vi "Factorial_Assignement.vi"() -> ()   [LabVIEW 2019]
panel:
  out "Result":i32
  in  "Numeric 2":i32
  # "Factorial Assignment"
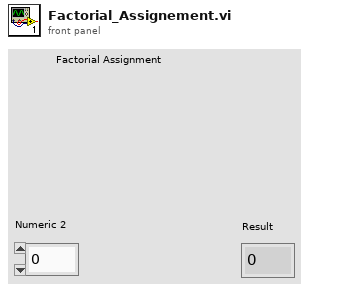
[diagram p1: front panel]
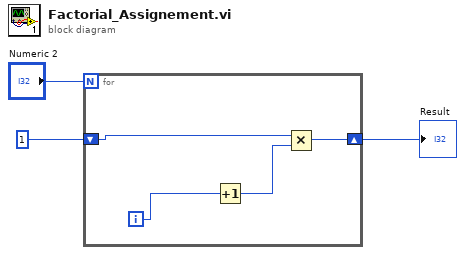
[diagram p0: block diagram]
diagram:
  n1 = for {
    N: "Numeric 2" -> [_]
    shift-right: [w4] -> w1
    shift-left: 1 -> [w7]
    i -> [w6]
    n2 = Increment(x=w6) -> (x+1=w5:i32)
    n3 = Multiply(x=w7, y=w5) -> (x*y=w4:i32)
  }
  "Result" <- w1
